vi "CHECK_Particular_SubCondition.vi"(7 "Reset?":bool, 9 "Specifier structure":T4, 10 "Current animal coordinates and stats":T5 {"Measurements and statistics"."Running, perc. of time" format="%05.2f"}, 11 "Frame length, ms":dbl) -> (3 "Valid?":bool)   [LabVIEW 2018, in "Tracker.lvlib"]
uses:
  Tracker.lvlib
  Controls/CTL_Full_data_frame.ctl
  Controls/CTL_Animal_Coordinates_and_Speed.ctl
  Controls/CTL_Measurements_and_Statistics.ctl
  Controls/CTL_Condition_type.ctl
  Controls/CTL_Comparison_type.ctl
  Controls/CTL_Validity_check_criteria.ctl
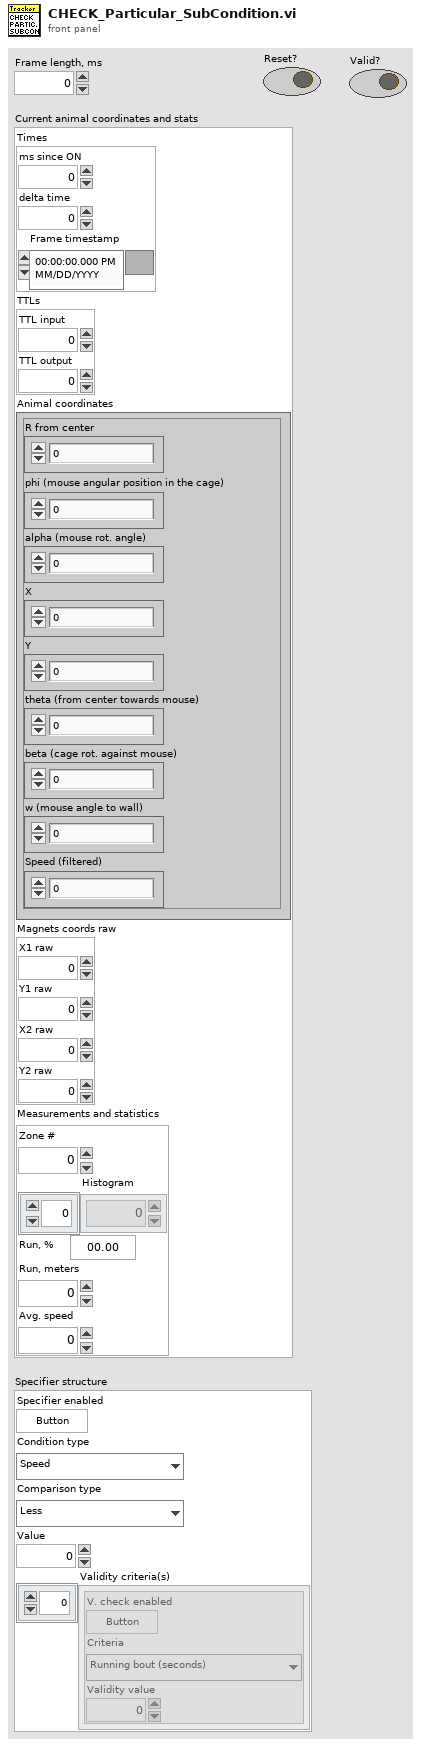
[diagram p1: front panel]
types:
  T1 = typedef "Tracker.lvlib/CTL_Condition_type.ctl" = enum16{"Speed", "Zone", "Angle to wall"}
  T2 = typedef "Tracker.lvlib/CTL_Comparison_type.ctl" = enum16{"Less", "Less or Equal", "Equal", "Greater or Equal", "Greater", "Not Equal"}
  T3 = typedef "Tracker.lvlib/CTL_Validity_check_criteria.ctl" = enum16{"Running bout (seconds)", "Running bout (meters)"}
  T4 = cluster{"Specifier enabled":bool, "Condition type":T1, "Comparison type":T2, "Value":dbl, "Validity criteria(s)":cluster{"V. check enabled":bool, "Criteria":T3, "Validity value":dbl}[]}
  T5 = typedef "Tracker.lvlib/CTL_Full_data_frame.ctl" = cluster{"Times":cluster{"ms since ON":u32, "delta time":u32, "Frame timestamp":timestamp}, "TTLs":cluster{"TTL input":i16, "TTL output":i16}, "Animal coordinates":T6, "Magnets coords raw":cluster{"X1 raw":dbl, "Y1 raw":dbl, "X2 raw":dbl, "Y2 raw":dbl}, "Measurements and statistics":T7}
  T6 = typedef "Tracker.lvlib/CTL_Animal_Coordinates_and_Speed.ctl" = cluster{"R from center":dbl, "phi (mouse angular position in the cage)":dbl, "alpha (mouse rot. angle)":dbl, "X":dbl, "Y":dbl, "theta (from center towards mouse)":dbl, "beta (cage rot. against mouse)":dbl, "w (mouse angle to wall)":dbl, "Speed (filtered)":dbl}
  T7 = typedef "Tracker.lvlib/CTL_Measurements_and_Statistics.ctl" = cluster{"Zone #":i8, "Histogram":dbl[], "Running, perc. of time":dbl, "Run, meters":dbl, "Avg. speed":dbl}
  T8 = cluster{"V. check enabled":bool, "Criteria":T3, "Validity value":dbl}[]
  T9 = cluster{"V. check enabled":bool, "Criteria":T3, "Validity value":dbl}
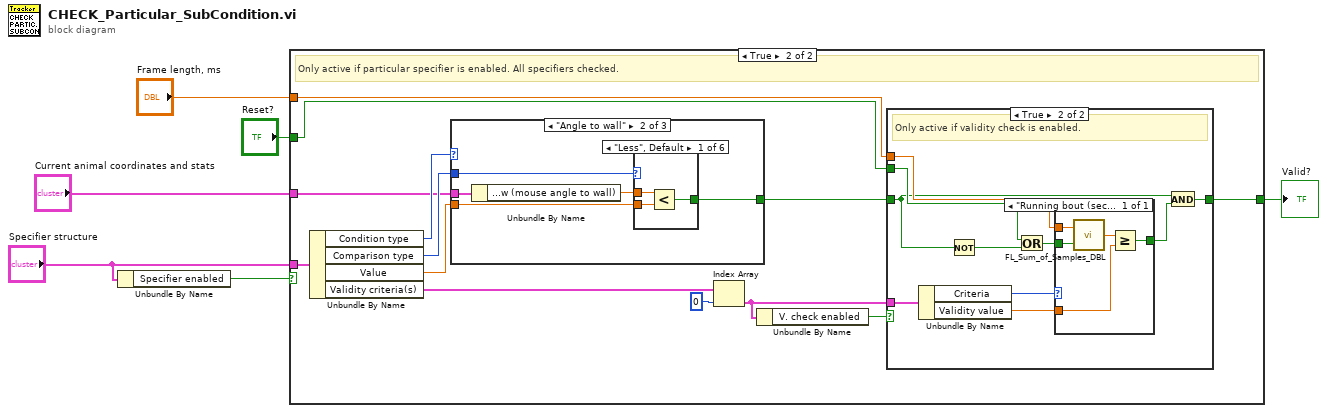
[diagram p0: block diagram]
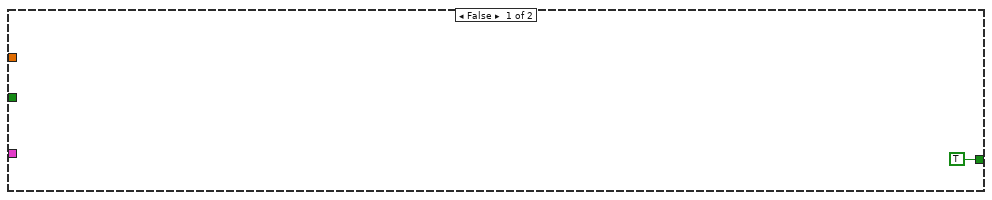
[diagram p2: hidden frame]
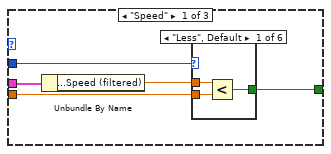
[diagram p3: hidden frame]
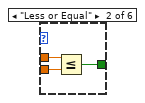
[diagram p4: hidden frame]
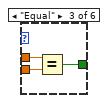
[diagram p5: hidden frame]
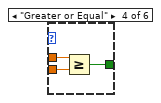
[diagram p6: hidden frame]
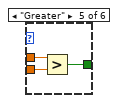
[diagram p7: hidden frame]
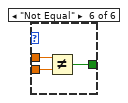
[diagram p8: hidden frame]
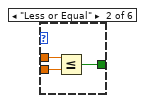
[diagram p9: hidden frame]
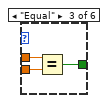
[diagram p10: hidden frame]
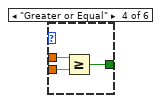
[diagram p11: hidden frame]
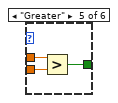
[diagram p12: hidden frame]
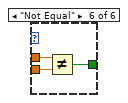
[diagram p13: hidden frame]
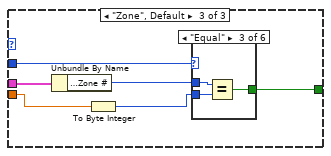
[diagram p14: hidden frame]
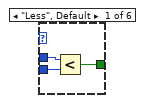
[diagram p15: hidden frame]
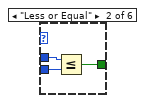
[diagram p16: hidden frame]
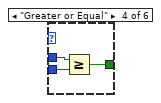
[diagram p17: hidden frame]
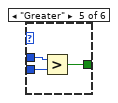
[diagram p18: hidden frame]
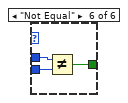
[diagram p19: hidden frame]
diagram:
  n1 = Unbundle By Name("Specifier structure") -> ("Specifier enabled"=w2:bool)
  n2 = case shown="True" w2 {
    tunnel: "Specifier structure" -> [_ w20]
    tunnel: [TRUE w9] -> w4
    tunnel: "Current animal coordinates and stats" -> [_ w12]
    tunnel: "Frame length, ms" -> [_ w10]
    tunnel: "Reset?" -> [_ w8]
    frame False {
    }
    frame True {
      # "Only active if particular specifier is enabled. All specifiers checked."
      n3 = Unbundle By Name(w20) -> ("Condition type"=w17:T1, "Comparison type"=w14:T2, "Value"=w15:dbl, "Validity criteria(s)"=w19:T8)
      n4 = case shown="\"Zone\", Default" w17 {
        tunnel: w12 -> [w25 w48 w72]
        tunnel: w15 -> [w23 w46 w70]
        tunnel: w14 -> [w22 w45 w69]
        tunnel: [w21 w44 w67] -> w11
        frame "Speed" {
          n5 = Unbundle By Name(w25) -> ("Animal coordinates.Speed (filtered)"=w24:dbl)
          n6 = case shown="\"Less\", Default" w22 {
            tunnel: w24 -> [w28 w31 w34 w37 w40 w43]
            tunnel: [w27 w30 w33 w36 w39 w42] -> w21
            tunnel: w23 -> [w26 w29 w32 w35 w38 w41]
            frame "Less", Default {
              n7 = Less?(x=w28, y=w26) -> (x < y?=w27:bool)
            }
            frame "Less or Equal" {
              n8 = Less Or Equal?(x=w31, y=w29) -> (x <= y?=w30:bool)
            }
            frame "Equal" {
              n9 = Equal?(x=w34, y=w32) -> (x = y?=w33:bool)
            }
            frame "Greater or Equal" {
              n10 = Greater Or Equal?(x=w37, y=w35) -> (x >= y?=w36:bool)
            }
            frame "Greater" {
              n11 = Greater?(x=w40, y=w38) -> (0:w39:bool)
            }
            frame "Not Equal" {
              n12 = Not Equal?(x=w43, y=w41) -> (x != y?=w42:bool)
            }
          }
        }
        frame "Angle to wall" {
          n13 = Unbundle By Name(w48) -> ("Animal coordinates.w (mouse angle to wall)"=w47:dbl)
          n14 = case shown="\"Less\", Default" w45 {
            tunnel: w47 -> [w51 w54 w57 w60 w63 w66]
            tunnel: [w50 w53 w56 w59 w62 w65] -> w44
            tunnel: w46 -> [w49 w52 w55 w58 w61 w64]
            frame "Less", Default {
              n15 = Less?(x=w51, y=w49) -> (x < y?=w50:bool)
            }
            frame "Less or Equal" {
              n16 = Less Or Equal?(x=w54, y=w52) -> (x <= y?=w53:bool)
            }
            frame "Equal" {
              n17 = Equal?(x=w57, y=w55) -> (x = y?=w56:bool)
            }
            frame "Greater or Equal" {
              n18 = Greater Or Equal?(x=w60, y=w58) -> (x >= y?=w59:bool)
            }
            frame "Greater" {
              n19 = Greater?(x=w63, y=w61) -> (0:w62:bool)
            }
            frame "Not Equal" {
              n20 = Not Equal?(x=w66, y=w64) -> (x != y?=w65:bool)
            }
          }
        }
        frame "Zone", Default {
          n21 = Unbundle By Name(w72) -> ("Measurements and statistics.Zone #"=w71:i8)
          n22 = To Byte Integer(number=w70) -> (8bit integer=w68:i8)
          n23 = case shown="\"Equal\"" w69 {
            tunnel: w71 -> [w75 w78 w81 w84 w87 w90]
            tunnel: [w74 w77 w80 w83 w86 w89] -> w67
            tunnel: w68 -> [w73 w76 w79 w82 w85 w88]
            frame "Less", Default {
              n24 = Less?(x=w75, y=w73) -> (x < y?=w74:bool)
            }
            frame "Less or Equal" {
              n25 = Less Or Equal?(x=w78, y=w76) -> (x <= y?=w77:bool)
            }
            frame "Equal" {
              n26 = Equal?(x=w81, y=w79) -> (x = y?=w80:bool)
            }
            frame "Greater or Equal" {
              n27 = Greater Or Equal?(x=w84, y=w82) -> (x >= y?=w83:bool)
            }
            frame "Greater" {
              n28 = Greater?(x=w87, y=w85) -> (0:w86:bool)
            }
            frame "Not Equal" {
              n29 = Not Equal?(x=w90, y=w88) -> (x != y?=w89:bool)
            }
          }
        }
      }
      n30 = Index Array(array=w19, index=0) -> (element=w13:T9)
      n31 = Unbundle By Name(w13) -> ("V. check enabled"=w16:bool)
      n32 = case shown="True" w16 {
        tunnel: w11 -> [w91 w93]
        tunnel: [w91 w98] -> w9
        tunnel: w13 -> [_ w101]
        tunnel: w10 -> [_ w96]
        tunnel: w8 -> [_ w95]
        frame False {
        }
        frame True {
          # "Only active if validity check is enabled."
          n33 = Unbundle By Name(w101) -> ("Criteria"=w100:T3, "Validity value"=w99:dbl)
          n34 = Not(x=w93) -> (.not. x?=w92:bool)
          n35 = Or(x=w95, y=w92) -> (x .or. y?=w94:bool)
          n36 = case shown="\"Running bout (seconds)\", Default" w100 {
            tunnel: w99 -> [w106]
            tunnel: w94 -> [w102]
            tunnel: [w105] -> w97
            tunnel: w96 -> [w104]
            frame "Running bout (seconds)", Default {
              n37 = call "FL_Sum_of_Samples_DBL.vi"("Reset?"=w102, "Input sample"=w104) -> ("Sum of samples"=w103:dbl)
              n38 = Greater Or Equal?(x=w103, y=w106) -> (x >= y?=w105:bool)
            }
          }
          n39 = And(x=w93, y=w97) -> (x .and. y?=w98:bool)
        }
      }
    }
  }
  "Valid?" <- w4
